vi "Convert Filter INI String to Cluster.vi"(11 "INI String":string) -> (3 "Filter Info":T1={"Filter Column"=enum."Description", "Filter Type"=enum."Contains", "Filter Value"="", "New Data?"=FALSE, "Case Sensitive?"=FALSE, "Enabled?"=FALSE})   [LabVIEW 2020, in "VI Properties Editor.lvlib"]
doc: "Converts a filter as <B>INI String</B> to a cluster."
uses:
  VI Properties Editor.lvlib
  CTLs/Filter Column.ctl
  CTLs/Filter Type.ctl
  CTLs/Filter Info.ctl
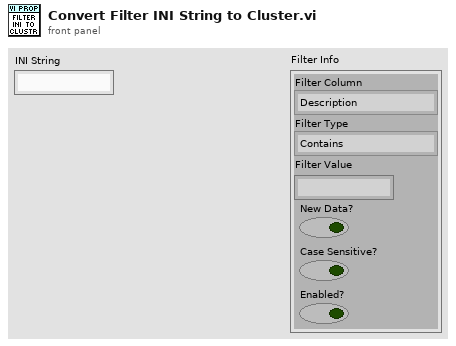
[diagram p1: front panel]
types:
  T1 = typedef "VI Properties Editor.lvlib/Filter Info.ctl" = cluster{"Filter Column":T2, "Filter Type":T3, "Filter Value":string, "New Data?":bool, "Case Sensitive?":bool, "Enabled?":bool}
  T2 = typedef "VI Properties Editor.lvlib/Filter Column.ctl" = enum16{"Name", "Path", "Type", "Window Title", "Description", "Help Path", "Help Tag", "Custom Title?", "Reentrancy", "Inlined?", "Help URL", "Help Type", "Allow Debugging?", "Auto Error Handling?", "Run When Opened?", "Suspend When Called?", "Priority", "Preferred Exec Sytem", "Control Label", "Control Caption", "Control Description", "Control Tip Strip"}
  T3 = typedef "VI Properties Editor.lvlib/Filter Type.ctl" = enum16{"Contains", "Equals", "Starts with", "Ends with", "Is empty", "Does not contain", "Does not equal", "Is not empty"}
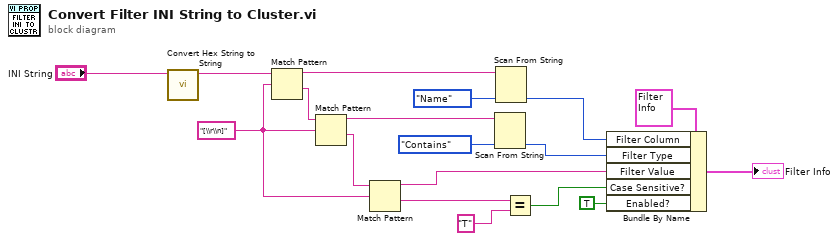
[diagram p0: block diagram]
diagram:
  w7 = "[\\r\\n]" ("regular expression")
  n1 = call "Convert Hex String to String.vi"("Hex String"="INI String") -> ("String"=w1:string)  [unwired: 10 in]
  n2 = Match Pattern(string=w1, regular expression=w7) -> (before substring=w16:string, after substring=w18:string)  [unwired: 1 in, 2 out]
  n3 = Match Pattern(string=w18, regular expression=w7) -> (before substring=w15:string, after substring=w8:string)  [unwired: 1 in, 2 out]
  n4 = Match Pattern(string=w8, regular expression=w7) -> (before substring=w6:string, after substring=w5:string)  [unwired: 1 in, 2 out]
  n5 = Scan From String(input string=w15, default 1=Filter_Type."Contains" ("Filter Type")) -> (output 1=w11:T3)  [unwired: 3 in, 3 out]
  n6 = Scan From String(input string=w16, default 1=Filter_Column."Name" ("Filter Column")) -> (output 1=w13:T2)  [unwired: 3 in, 3 out]
  n7 = Equal?(x=w5, y="T") -> (x = y?=w3:bool)
  n8 = Bundle By Name(cluster=T1 {"Filter Column"=enum."Description", "Filter Type"=enum."Contains", "Filter Value"="", "New Data?"=FALSE, "Case Sensitive?"=FALSE, "Enabled?"=FALSE} ("Filter Info"), "Filter Column"=w13, "Filter Type"=w11, "Filter Value"=w6, "Case Sensitive?"=w3, "Enabled?"=TRUE) -> (→"Filter Info":T1)
